vi "Read_ADS1100_2.vi"(2 "error in (no error)":errorcluster, 3 "USB DAQ Address":i32 format="%x", 4 "ADS Mode":i32, 5 "ADS number":i32=1) -> (0 "error out":errorcluster, 1 "ADC":dbl)   [LabVIEW 2011]
doc: "This is a wrapper VI for the \"tio32_read_ADS1100\" VI by LPSE. It behaves exactly the same as that VI, except it also converts the ADC number and ADC voltages into strings which are then output to the global string variable which is used to populate the \"TI Debug Window\" VI."
uses:
  INA231/Global Variables.vi
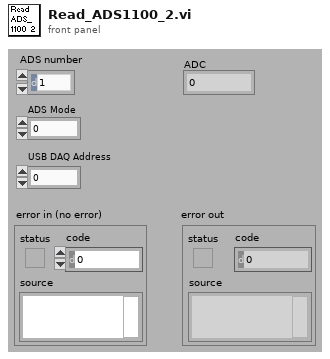
[diagram p1: front panel]
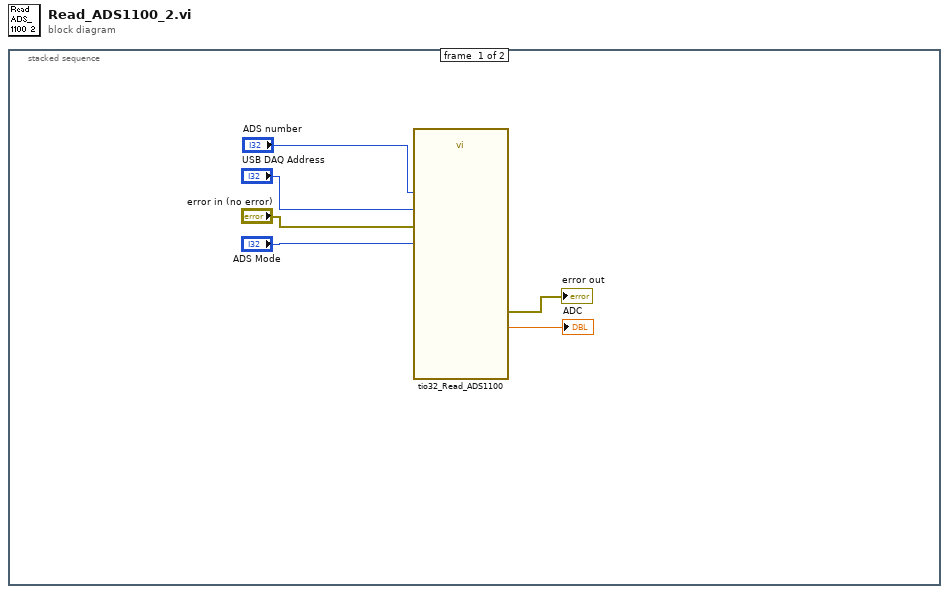
[diagram p0: block diagram]
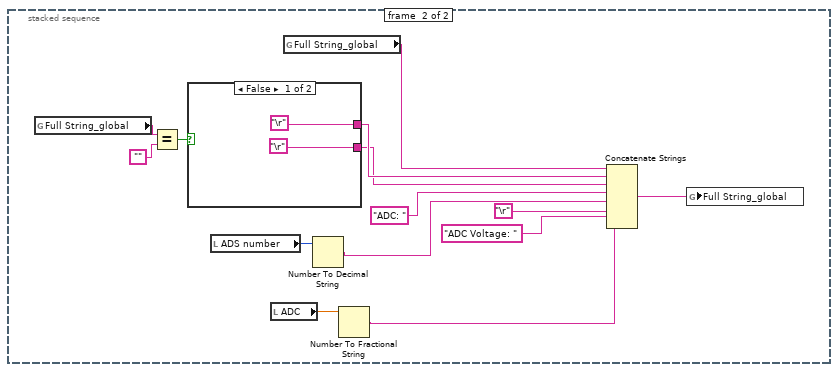
[diagram p2: hidden frame]
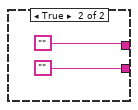
[diagram p3: hidden frame]
diagram:
  n1 = stacked-sequence {
    frame #0 {
      n2 = call "tio32_Read_ADS1100.vi"("Board address"="USB DAQ Address", "ADS number"="ADS number", "mode"="ADS Mode", "error in (no error)"="error in (no error)") -> ("value"=→"ADC":dbl, "error out"=→"error out":errorcluster)  [unwired: 7 in, 3 out]
    }
    frame #1 {
      n3 = global read "Global Variables.vi" "Full String_global"() -> (w19:string)
      n4 = Equal?(x=w19, y="") -> (x = y?=w20:bool)
      n5 = case shown="False" w20 {
        tunnel: ["\r" ""] -> w15
        tunnel: ["\r" ""] -> w14
        frame False {
        }
        frame True {
        }
      }
      n6 = local read "ADS number"() -> (w7:i32)
      n7 = local read "ADC"() -> (w9:dbl)
      n8 = global read "Global Variables.vi" "Full String_global"() -> (w16:string)
      n9 = Number To Decimal String(number=w7) -> (decimal integer string=w8:string)  [unwired: 1 in]
      n10 = Number To Fractional String(number=w9) -> (F-format string=w10:string)  [unwired: 3 in]
      n11 = Concatenate Strings(w16, w15, w14, "ADC: ", w8, "\r", "ADC Voltage: ", w10) -> (w17:string)
      n12 = global write "Global Variables.vi" "Full String_global"(w17) -> ()
    }
  }
